vi "Check rake lines.vi"(10 "Angle info (Process)":T1, 11 "Angle info (Template)":T1) -> (2 "Angle info (Process)":T1, 3 "Angle info (Template)":T1)   [LabVIEW 2015]
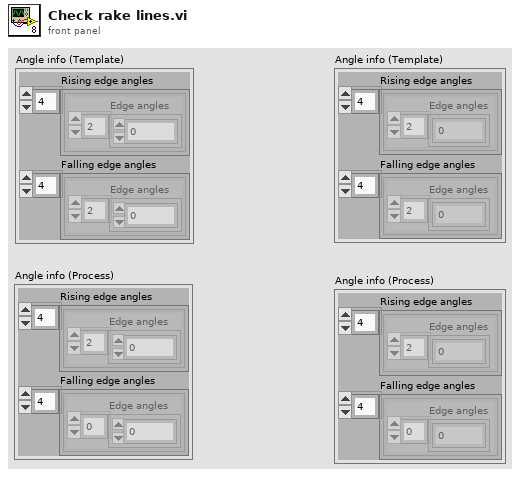
[diagram p1: front panel]
types:
  T1 = cluster{"Rising edge angles":cluster{"Edge angles":dbl[]}[], "Falling edge angles":cluster{"Edge angles":dbl[]}[]}
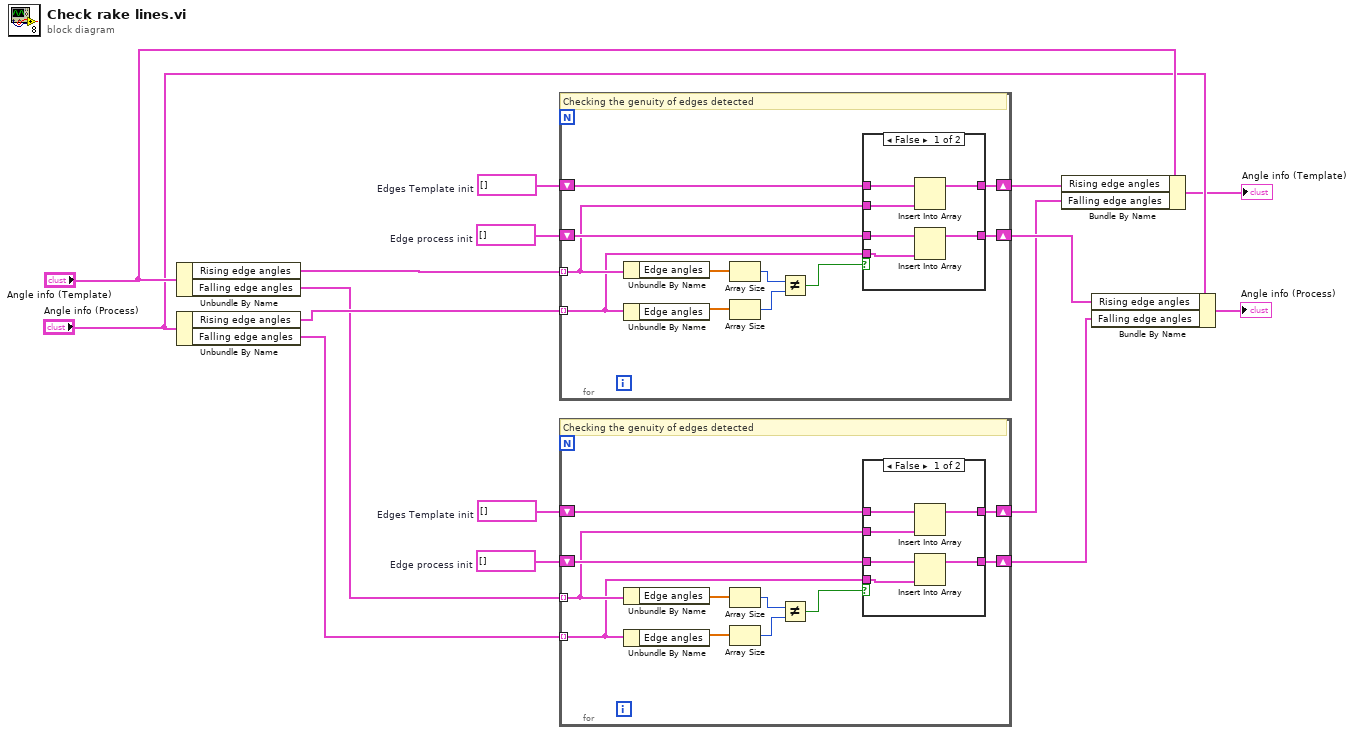
[diagram p0: block diagram]
diagram:
  w13 = cluster{"Edge angles":dbl[]}[] []  # Edges Template init
  w14 = cluster{"Edge angles":dbl[]}[] []  # Edge process init
  w16 = cluster{"Edge angles":dbl[]}[] []  # Edges Template init
  w15 = cluster{"Edge angles":dbl[]}[] []  # Edge process init
  n1 = Unbundle By Name("Angle info (Template)") -> ("Rising edge angles"=w12:cluster{"Edge angles":dbl[]}[], "Falling edge angles"=w10:cluster{"Edge angles":dbl[]}[])
  n2 = Unbundle By Name("Angle info (Process)") -> ("Rising edge angles"=w11:cluster{"Edge angles":dbl[]}[], "Falling edge angles"=w9:cluster{"Edge angles":dbl[]}[])
  n3 = for {
    tunnel: w12 -> [w20] mode=indexing
    tunnel: w11 -> [w19] mode=indexing
    shift-right: [w18] -> w6
    shift-left: w16 -> [w23]
    shift-right: [w17] -> w5
    shift-left: w15 -> [w22]
    # "Checking the genuity of edges detected"
    n4 = Unbundle By Name(w20) -> ("Edge angles"=w24:dbl[])
    n5 = Unbundle By Name(w19) -> ("Edge angles"=w25:dbl[])
    n6 = Array Size(array=w24) -> (size(s)=w27:i32)
    n7 = Array Size(array=w25) -> (size(s)=w26:i32)
    n8 = Not Equal?(x=w27, y=w26) -> (x != y?=w21:bool)
    n9 = case shown="False" w21 {
      tunnel: w23 -> [w33 w35]
      tunnel: w22 -> [w32 w34]
      tunnel: w20 -> [w31 _]
      tunnel: w19 -> [w30 _]
      tunnel: [w29 w35] -> w18
      tunnel: [w28 w34] -> w17
      frame False {
        n10 = Insert Into Array(array=w33, new element=w31) -> (w29:cluster{"Edge angles":dbl[]}[])  [unwired: 1 in]
        n11 = Insert Into Array(array=w32, new element=w30) -> (w28:cluster{"Edge angles":dbl[]}[])  [unwired: 1 in]
      }
      frame True {
      }
    }
  }
  n12 = for {
    tunnel: w10 -> [w39] mode=indexing
    tunnel: w9 -> [w38] mode=indexing
    shift-right: [w37] -> w4
    shift-left: w13 -> [w42]
    shift-right: [w36] -> w3
    shift-left: w14 -> [w41]
    # "Checking the genuity of edges detected"
    n13 = Unbundle By Name(w39) -> ("Edge angles"=w43:dbl[])
    n14 = Unbundle By Name(w38) -> ("Edge angles"=w44:dbl[])
    n15 = Array Size(array=w43) -> (size(s)=w46:i32)
    n16 = Array Size(array=w44) -> (size(s)=w45:i32)
    n17 = Not Equal?(x=w46, y=w45) -> (x != y?=w40:bool)
    n18 = case shown="False" w40 {
      tunnel: w42 -> [w52 w54]
      tunnel: w41 -> [w51 w53]
      tunnel: w39 -> [w50 _]
      tunnel: w38 -> [w49 _]
      tunnel: [w48 w54] -> w37
      tunnel: [w47 w53] -> w36
      frame False {
        n19 = Insert Into Array(array=w52, new element=w50) -> (w48:cluster{"Edge angles":dbl[]}[])  [unwired: 1 in]
        n20 = Insert Into Array(array=w51, new element=w49) -> (w47:cluster{"Edge angles":dbl[]}[])  [unwired: 1 in]
      }
      frame True {
      }
    }
  }
  n21 = Bundle By Name(cluster="Angle info (Template)", "Rising edge angles"=w6, "Falling edge angles"=w4) -> (→"Angle info (Template)":T1)
  n22 = Bundle By Name(cluster="Angle info (Process)", "Rising edge angles"=w5, "Falling edge angles"=w3) -> (→"Angle info (Process)":T1)
